vi "TempControl.vi"() -> ()   [LabVIEW 2014]
panel:
  out "Thermometer":dbl(slide) scale=0.0..100.0
  in  "Manual/Auto":bool
  in  "Heater":bool
  in  "AC":bool
  out "Manual":bool
  out "Heat":bool
  out "AC":bool
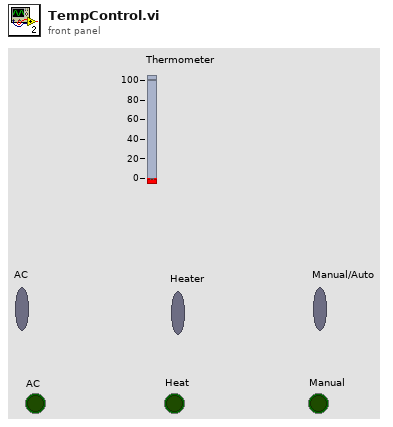
[diagram p1: front panel]
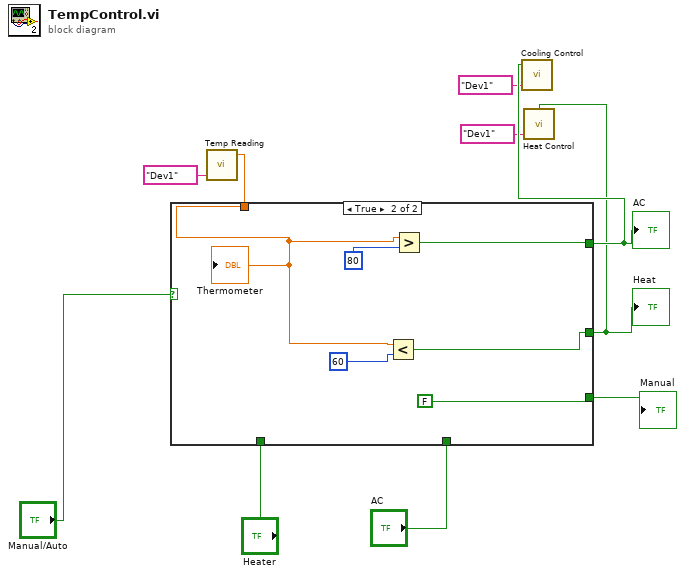
[diagram p0: block diagram]
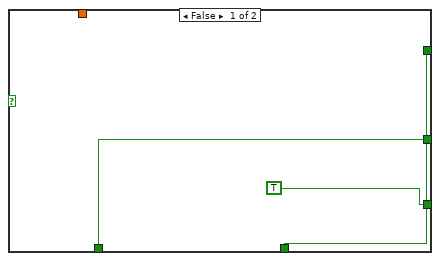
[diagram p2: hidden frame]
diagram:
  n1 = call "Temp Reading.vi"("device name"=tag "Dev1") -> ("Result"=w6:dbl)  [unwired: 1 in]
  n2 = case shown="True" "Manual/Auto" {
    tunnel: [TRUE FALSE] -> w10
    tunnel: [w11 w16] -> w5
    tunnel: [w12 w15] -> w4
    tunnel: "Heater" -> [w12 _]
    tunnel: "AC" -> [w11 _]
    tunnel: w6 -> [_ w14]
    frame False {
    }
    frame True {
      n3 = Less?(x=w14, y=60) -> (x < y?=w15:bool)
      n4 = Greater?(x=w14, y=80) -> (0:w16:bool)
      "Thermometer" <- w14
    }
  }
  "AC" <- w5
  "Heat" <- w4
  "Manual" <- w10
  n5 = call "Cooling Control.vi"("Device Name"=tag "Dev1", "Cooling"=w5) -> ()  [unwired: 1 in]
  n6 = call "Heat Control.vi"("device name"=tag "Dev1", "Heat"=w4) -> ()  [unwired: 1 in]
